vi "Execute Query.vi"(6 "Config Query in":refnum<class "CConfig Query.lvclass">, 8 "error in (no error)":errorcluster, 11 "Carya Config in":refnum<class "Carya Config.lvclass">) -> (0 "error out":errorcluster, 1 "Results":string[][](array[string]), 2 "Result":bool, 3 "Carya Config out":refnum<class "Carya Config.lvclass">, 4 "Index":i32)   [LabVIEW 2013, in "Carya Config.lvclass"]
doc: "Copyright 2018, Carya Automatisering, Wiebe Walstra."
uses:
  Carya Config.lvclass
  CConfig Object/CConfig Query.lvclass
  Carya Config.lvclass/Carya Config.ctl
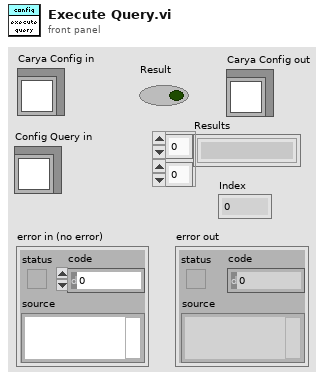
[diagram p1: front panel]
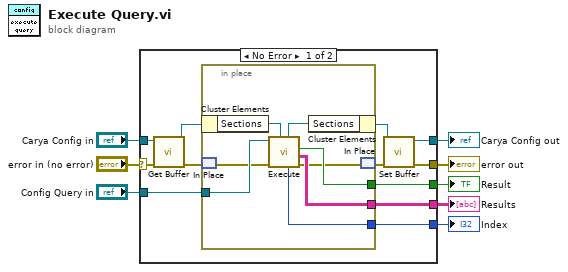
[diagram p0: block diagram]
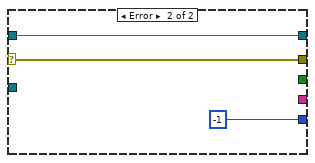
[diagram p2: hidden frame]
diagram:
  n1 = case shown="No Error" "error in (no error)" {
    selector: "error in (no error)" -> [w20 w31]
    tunnel: [w17 w31] -> w7
    tunnel: [w16 w30] -> w5
    tunnel: "Carya Config in" -> [w18 w30]
    tunnel: [w19 _] -> w4
    tunnel: "Config Query in" -> [w13 _]
    tunnel: [w12 -1 ("Index")] -> w2
    tunnel: [w11 _] -> w1
    frame No Error {
      n2 = call-dynamic "Get Buffer.vi"("error in (no error)"=w20, "Carya Config in"=w18) -> ("error out"=w10:errorcluster, "Config"=w15:refnum<class "Carya Config.lvclass">)  [unwired: 8 in]
      n3 = in-place {
        in-place-border: [w26] -> w19
        in-place-border: w13 -> [w25]
        in-place-border: [w24] -> w12
        in-place-border: [w23] -> w11
        n4 = in-place-cluster #1(w15) -> ("Sections"=w28:refnum<class "CConfig Object.lvclass">)
        n5 = in-place-match #2(w10) -> (w22:errorcluster)
        n6 = call-dynamic "Execute.vi"("Composite Object"=w28, "error in (no error)"=w22, "Config Query in"=w25) -> ("error out"=w21:errorcluster, "Results"=w26:string[][], "Result"=w23:bool, "Index"=w24:i32, "Composite Object"=w27:refnum<class "CConfig Object.lvclass">)  [unwired: 3 in, 1 out]
        n7 = in-place-cluster #1("Sections"=w27) -> (w14:refnum<class "Carya Config.lvclass">)
        n8 = in-place-match #2(w21) -> (w9:errorcluster)
      }
      n9 = call-dynamic "Set Buffer.vi"("error in (no error)"=w9, "Carya Config"=w14) -> ("error out"=w17:errorcluster, "Carya Config out"=w16:refnum<class "Carya Config.lvclass">)  [unwired: 8 in]
    }
    frame Error {
    }
  }
  "error out" <- w7
  "Carya Config out" <- w5
  "Results" <- w4
  "Index" <- w2
  "Result" <- w1
